vi "calculate level.vi"(8 "error in (no error)":errorcluster, 11 "device queue":refnum<class "Message Enqueuer.lvclass">) -> (0 "error out":errorcluster)   [LabVIEW 2020, in "calibration.lvlib"]
uses:
  calibration.lvlib
  calibration Messages/calculate level Msg/calculate level Msg.lvclass
  <vilib>/ActorFramework/Message Enqueuer/Message Enqueuer.lvclass
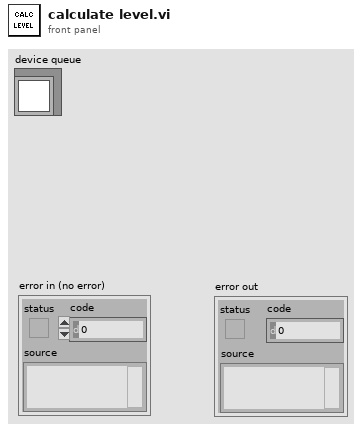
[diagram p1: front panel]
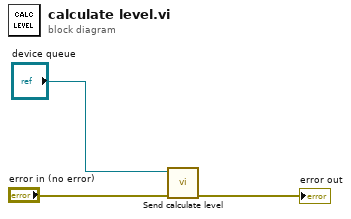
[diagram p0: block diagram]
diagram:
  n1 = call "Send calculate level.vi"("error in (no error)"="error in (no error)", "Message Enqueuer"="device queue") -> ("error out"=→"error out":errorcluster)  [unwired: 8 in, 1 out]
